vi "MainVI.vi"() -> ()   [LabVIEW 2015]
uses:
  <vilib>/imath/engines/lvmath/Plug In/_Char/NIMS_CH_character datatype.ctl
  <vilib>/myRIO/Instrument Drivers/Onboard IO/UART/typedef/VISA Configuration.ctl
  <vilib>/myRIO/Common/Instrument Driver Framework/myRIO v1.0/UART/vis/myRIO v1.0 Close UART.vi
  <vilib>/imath/engines/lvmath/Plug In/_Char/NIMS_CH_Character RV to String.vi
  <vilib>/imath/engines/lvmath2/RunTimeEngine/NodeEndStatement/NIMS_NodeEndStatement_Output.vi
  <instcachedir>/0/NIMS_NodeEndStatement_Output_53EC0D466D134D7ABD903AC30B43404B.lvgen/NIMS_NodeEndStatement_Output_53EC0D466D134D7ABD903AC30B43404B_008.vi
  <vilib>/imath/engines/lvmath2/RunTimeEngine/ErrorHandling/NIMS_Finalize Error.vi
  <vilib>/Instr/_visa.llb/VISA Configure Serial Port (Instr).vi
  <vilib>/myRIO/Common/Instrument Driver Framework/Utilities/vis/FPGA Ref Manager.vi
  <vilib>/myRIO/Common/Instrument Driver Framework/myRIO v1.0/myRIO v1.0 Reset FPGA.vi
  <vilib>/myRIO/Common/Instrument Driver Framework/myRIO v1.0/IRQ/vis/myRIO v1.0 IRQ Info FGV.vi
  <vilib>/myRIO/Common/Instrument Driver Framework/myRIO v1.0/IRQ/vis/myRIO v1.0 Timer IRQ Info FGV.vi
  <vilib>/myRIO/Common/Instrument Driver Framework/myRIO v1.0/IRQ/vis/myRIO v1.0 ISR Agent.vi
  <vilib>/myRIO/Express VI/Onboard IO/UART/UART Express VI.xnode
  <vilib>/myRIO/Instrument Drivers/Utilities/Utilities.lvlib
  <vilib>/myRIO/Instrument Drivers/Onboard IO/UART/UART.lvlib
panel:
  out "Caracter":string
  out "y":sgl
  out "x":sgl
  out "Matches":dbl
  in  "Objeto a Reconocer":i16(slide)=1 min=1 max=3 scale=1.0..3.0
  out "Imagen Binarizada":T1(plugin-control)
  in  "stop":bool
  out "Imagen sin Procesamiento":T1(plugin-control)
  # "Proyecto Final de Sistemas de Innovación. NI Vision.  (Noviembre 2017)"
  # "Triángulo"
  # "'L'"
  # "Recta"
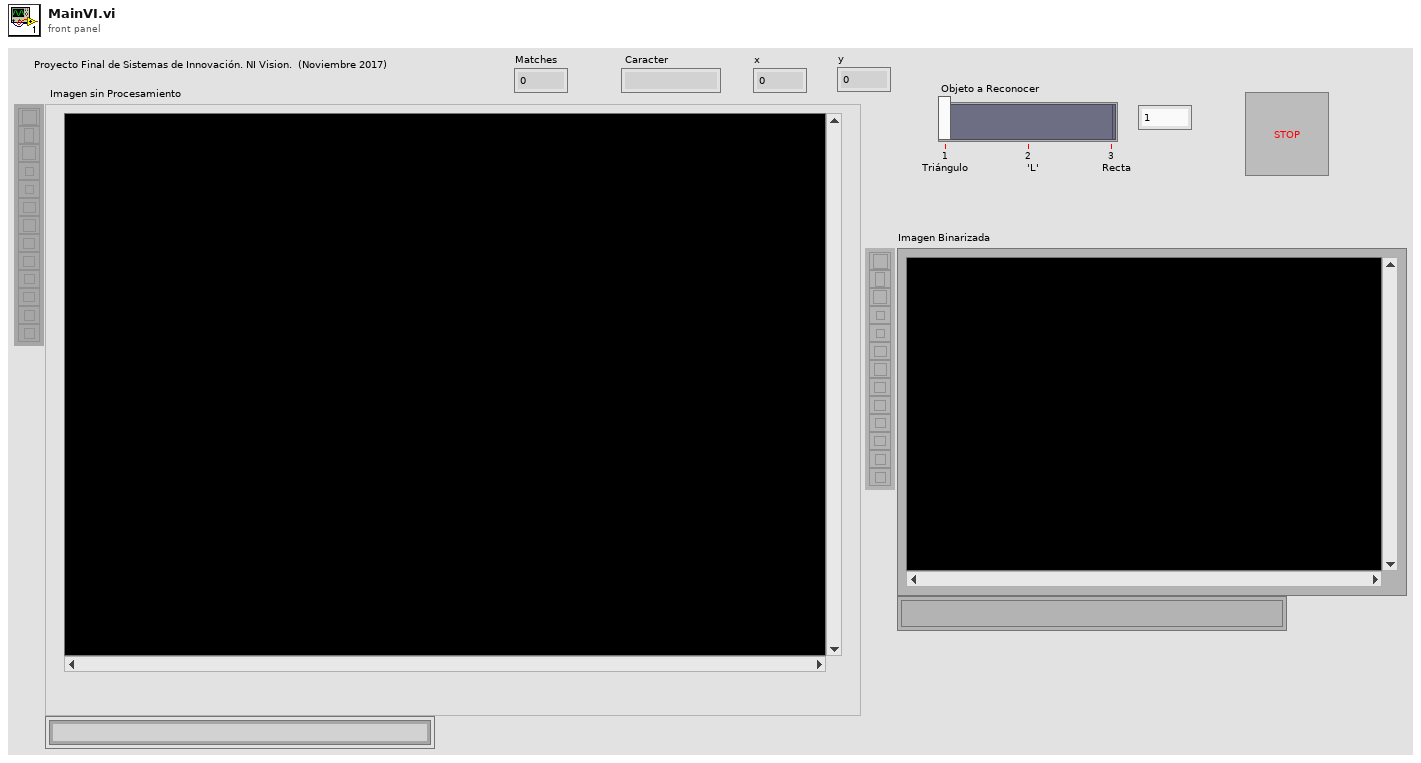
[diagram p1: front panel]
types:
  T1 = typedef "IMAQ Image.ctl" = refnum<image>
  T2 = typedef "UART.lvlib/VISA Configuration.ctl" = cluster{"baud rate (9600)":u32, "data bits (8)":u16, "parity (0:none)":enum16{"None", "Odd", "Even", "Mark", "Space"}, "stop bits (10: 1 bit)":u16, "flow control (0:none)":u16, "termination char\n(0xA = '\\n' = LF) ":u8, "Enable Termination\nChar (T)":bool, "timeout (10sec)":u32}
  T3 = typedef "NIMS_CH_character datatype.ctl" = cluster{"Numeric":u8}
  T4 = cluster{"Global Rectangle":cluster{"x1Left":i32, "y1Top":i32, "x2Right":i32, "y2Bottom":i32}, "Centroid":cluster{"x":sgl, "y":sgl}, "Object Size":u32, "Score":dbl}[]
  T5 = cluster{"Global Rectangle":cluster{"x1Left":i32, "y1Top":i32, "x2Right":i32, "y2Bottom":i32}, "Centroid":cluster{"x":sgl, "y":sgl}, "Object Size":u32, "Score":dbl}
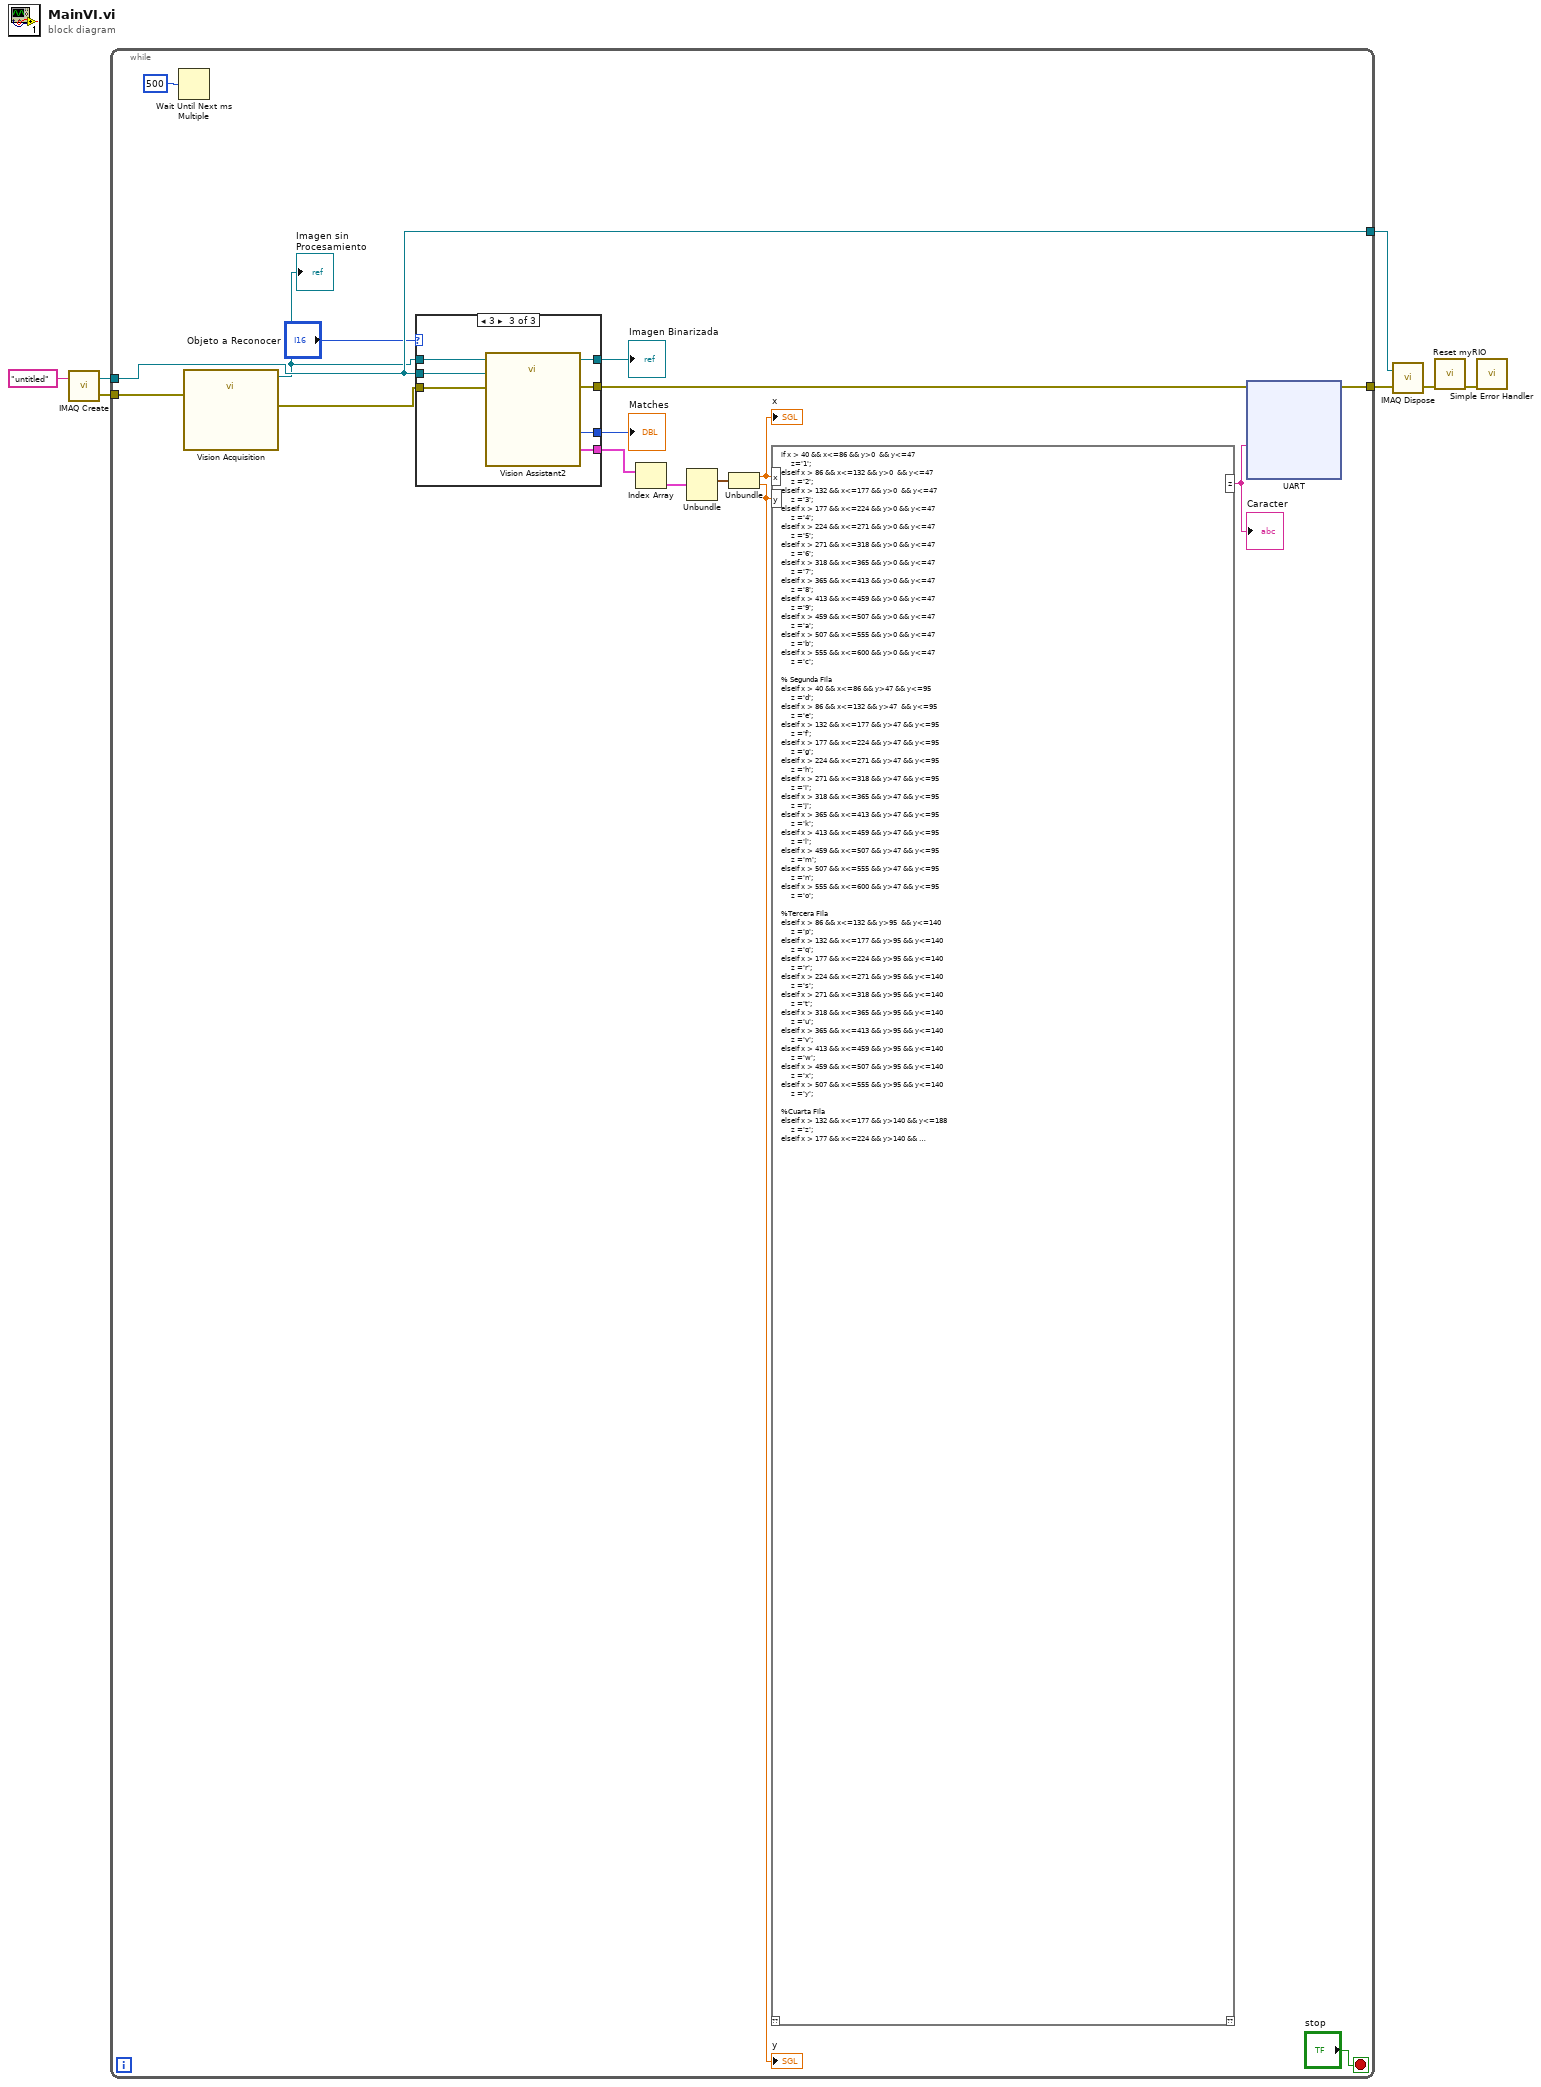
[diagram p0: block diagram]
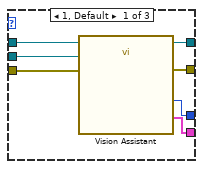
[diagram p2: hidden frame]
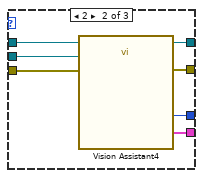
[diagram p3: hidden frame]
diagram:
  n1 = call "IMAQ Create"("Image Name"="untitled") -> ("New Image"=w3:T1, "error out"=w5:errorcluster)  [unwired: 4 in]
  n2 = while {
    tunnel: w5 -> [w23]
    tunnel: w3 -> [w22]
    tunnel: [w22] -> w2
    tunnel: [w11] -> w1
    stop <- "stop" stop-if-true
    n3 = Wait Until Next ms Multiple(millisecond multiple=u32 500) -> ()  [unwired: 1 out]
    n4 = call "Vision Acquisition"("error in"=w23) -> ("Image Out"=w21:T1, "error out"=w8:errorcluster)  [unwired: 25 in]
    "Imagen sin Procesamiento" <- w21
    n5 = case shown="3" "Objeto a Reconocer" {
      tunnel: w8 -> [w2042 w2045 w2054]
      tunnel: [w2041 w2048 w2053] -> w12
      tunnel: w22 -> [w2040 w2046 w2055]
      tunnel: w21 -> [w2039 w2047 w2056]
      tunnel: [w2038 w2049 w2052] -> w19
      tunnel: [w2037 w2044 w2051] -> w18
      tunnel: [w2036 w2043 w2050] -> w17
      frame 1, Default {
        n6 = call "Vision Assistant"("Image In"=w2039, "Image Dst"=w2040, "error in"=w2042) -> ("Image Out"=w2038:T1, "Number of Matches (Shape Matching 1)"=w2037:i32, "Shape Report (Shape Matching 1)"=w2036:T4, "error out"=w2041:errorcluster)  [unwired: 21 in]
      }
      frame 2 {
        n7 = call "Vision Assistant4"("Image In"=w2047, "Image Dst"=w2046, "error in"=w2045) -> ("Image Out"=w2049:T1, "Number of Matches (Shape Matching 1)"=w2044:i32, "Shape Report (Shape Matching 1)"=w2043:T4, "error out"=w2048:errorcluster)  [unwired: 21 in]
      }
      frame 3 {
        n8 = call "Vision Assistant2"("Image In"=w2056, "Image Dst"=w2055, "error in"=w2054) -> ("Image Out"=w2052:T1, "Number of Matches (Shape Matching 1)"=w2051:i32, "Shape Report (Shape Matching 1)"=w2050:T4, "error out"=w2053:errorcluster)  [unwired: 21 in]
      }
    }
    "Imagen Binarizada" <- w19
    "Matches" <- w18
    n9 = Index Array(array=w17) -> (element=w16:T5)  [unwired: 1 in]
    n10 = Unbundle(w16) -> ("Centroid"=w15:cluster{"x":sgl, "y":sgl})  [unwired: 3 out]
    n11 = Unbundle(w15) -> ("x"=w14:sgl, "y"=w13:sgl)
    "x" <- w14
    "y" <- w13
    n12 = mathscript code="if x > 40 && x<=86 && y>0  && y<=47\n     z='1';\nelseif x > 86 && x<=132 && y>0  && y<=47\n     z ='2';\nelseif x > 132 && x<=177 && y>0  && y<=47\n     z ='3';\nelseif x > 177 && x<=224 && y>0 && y<=47\n     z ='4';\nelseif x > 224 && x<=271 && y>0 && y<=47\n     z ='5';\nelseif x > 271 && x<=318 && y>0 && y<=47\n     z ='6';\nelseif x > 318 && x<=365 && y>0 && y<=47\n     z ='7';\nelseif x > 365 && x<=413 && y>0 && y<=47\n     z ='8';\nelseif x > 413 && x<=459 && y>0 && y<=47\n     z ='9';\nelseif x > 459 && x<=507 && y>0 && y<=47\n     z ='a';\nelseif x > 507 && x<=555 && y>0 && y<=47\n     z ='b';\nelseif x > 555 && x<=600 && y>0 && y<=47\n     z ='c';\n\n% Segunda Fila\nelseif x > 40 && x<=86 && y>47 && y<=95\n     z ='d';\nelseif x > 86 && x<=132 && y>47  && y<=95\n     z ='e';\nelseif x > 132 && x<=177 && y>47 && y<=95\n     z ='f';\nelseif x > 177 && x<=224 && y>47 && y<=95\n     z ='g';\nelseif x > 224 && x<=271 && y>47 && y<=95\n     z ='h';\nelseif x > 271 && x<=318 && y>47 && y<=95\n     z ='i';\nelseif x > 318 && x<=365 && y>47 && y<=95\n     z ='j';\nelseif x > 365 && x<=413 && y>47 && y<=95\n     z ='k';\nelseif x > 413 && x<=459 && y>47 && y<=95\n     z ='l';\nelseif x > 459 && x<=507 && y>47 && y<=95\n     z ='m';\nelseif x > 507 && x<=555 && y>47 && y<=95\n     z ='n';\nelseif x > 555 && x<=600 && y>47 && y<=95\n     z ='o';\n\n%Tercera Fila\nelseif x > 86 && x<=132 && y>95  && y<=140\n     z ='p';\nelseif x > 132 && x<=177 && y>95 && y<=140\n     z ='q';\nelseif x > 177 && x<=224 && y>95 && y<=140\n     z ='r';\nelseif x > 224 && x<=271 && y>95 && y<=140\n     z ='s';\nelseif x > 271 && x<=318 && y>95 && y<=140\n     z ='t';\nelseif x > 318 && x<=365 && y>95 && y<=140\n     z ='u';\nelseif x > 365 && x<=413 && y>95 && y<=140\n     z ='v';\nelseif x > 413 && x<=459 && y>95 && y<=140\n     z ='w';\nelseif x > 459 && x<=507 && y>95 && y<=140\n     z ='x';\nelseif x > 507 && x<=555 && y>95 && y<=140\n     z ='y';\n\n%Cuarta Fila\nelseif x > 132 && x<=177 && y>140 && y<=188\n     z ='z';\nelseif x > 177 && x<=224 && y>140 && y<=188\n     z ='!';\nelseif x > 224 && x<=271 && y>140 && y<=188\n     z ='\"';\nelseif x > 271 && x<=318 && y>140 && y<=188\n     z ='#';\nelseif x > 318 && x<=365 && y>140 && y<=188\n     z ='$';\nelseif x > 365 && x<=413 && y>140 && y<=188\n     z ='%';\nelseif x > 413 && x<=459 && y>140 && y<=188\n     z ='&';\nelseif x > 459 && x<=507 && y>140 && y<=188\n     z ='(';\n\n%Quinta Fila\nelseif x > 224 && x<=271 && y>188 && y<=235\n     z =')';\nelseif x > 271 && x<=318 && y>188 && y<=235\n     z ='*';\nelseif x > 318 && x<=365 && y>188 && y<=235\n     z ='-';\nelseif x > 365 && x<=413 && y>188 && y<=235\n     z ='/';\n\nelse\n    z ='0' ;\nend"("x"=w14, "y"=w13) -> ("z"=w10:string)  [unwired: 1 in, 1 out]
    "Caracter" <- w10
    n13 = xnode "UART"("Characters to Write"=w10, "error in (no error)"=w12) -> ("error out"=w11:errorcluster)  [unwired: 1 out]
  }
  n14 = call "IMAQ Dispose"("Image"=w2, "error in (no error)"=w1) -> ("error out"=w4:errorcluster)  [unwired: 4 in]
  n15 = call <vilib>:"Reset myRIO.vi"("error in (no error)"=w4) -> ("error out"=w7:errorcluster)  [unwired: 10 in]
  n16 = call <vilib>:"Simple Error Handler.vi"("error in (no error)"=w7) -> ()  [unwired: 4 in, 5 out]
